vi "YKMW100 Get Error Log.vi"(0 "VISA session":refnum<visa-resource-name>="MW100", 2 "Semiphore":T1, 9 "Timeout (25000)":u32=100, 11 "error in (no error)":errorcluster, 13 "Source (\"\")":string) -> (4 "dup VISA session":refnum<visa-resource-name>, 6 "Error History":string[](array[string]), 7 "Send Message (\"\")":string, 15 "error out":errorcluster)   [LabVIEW 2009]
doc: "This VI sends the message. Then it returns the response."
panel:
  out "Read Buffer":string
  in  "Number of Read Blocks (1-50)":i32
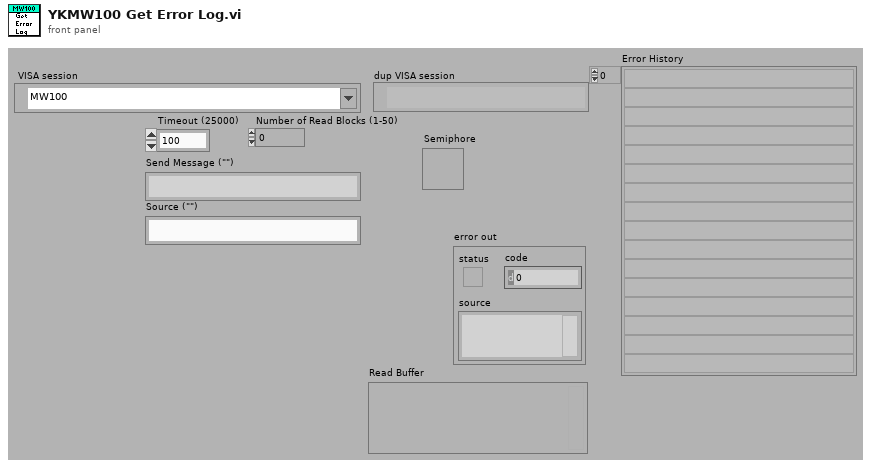
[diagram p1: front panel]
types:
  T1 = typedef "Semaphore RefNum" = refnum<k1>
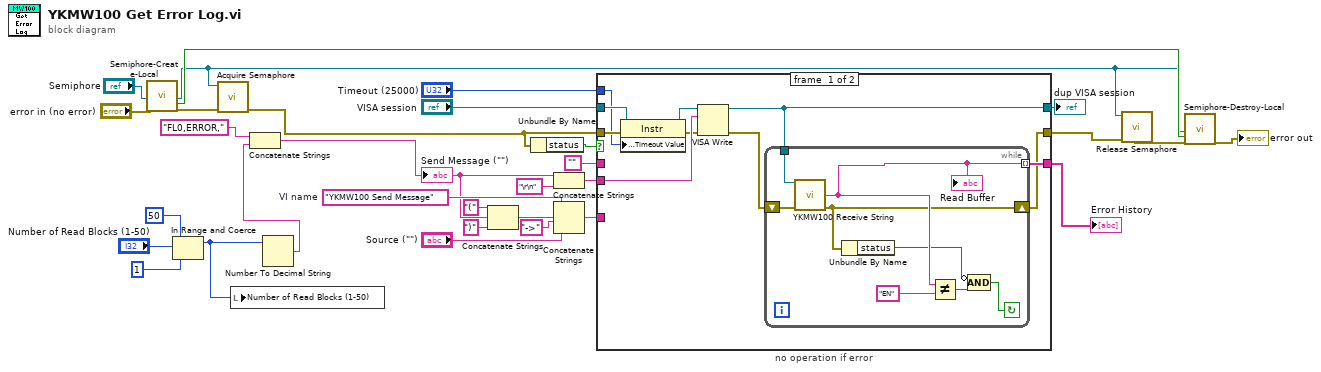
[diagram p0: block diagram]
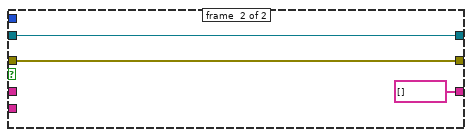
[diagram p2: hidden frame]
diagram:
  w21 = "YKMW100 Send Message"  # VI name
  n1 = call "Semiphore-Create-Local.vi"("Semiphore"="Semiphore", "error in (no error)"="error in (no error)") -> ("semaphore"=w1:T1, "Local?"=w4:bool, "error out"=w7:errorcluster)  [unwired: 15 in]
  n2 = In Range and Coerce(upper limit=50, x="Number of Read Blocks (1-50)", lower limit=1) -> (coerced(x)=w13:i32)  [unwired: 1 out]
  n3 = call <vilib>:"Acquire Semaphore.vi"("error in (no error)"=w7, "semaphore"=w1) -> ("error out"=w3:errorcluster)  [unwired: 3 in, 2 out]
  n4 = local write "Number of Read Blocks (1-50)"(w13) -> ()
  n5 = Number To Decimal String(number=w13) -> (decimal integer string=w12:string)  [unwired: 1 in]
  n6 = Concatenate Strings("FL0,ERROR,", w12) -> (w11:string)
  "Send Message (\"\")" <- w11
  n7 = Concatenate Strings("(", w11, ")") -> (w22:string)
  n8 = Unbundle By Name(w3) -> ("status"=w28:bool)
  n9 = Concatenate Strings(w11, "\r\n") -> (w31:string)
  n10 = Concatenate Strings(w21, w22, "->", "Source (\"\")") -> (w27:string)
  n11 = case "no operation if error" shown="False" w28 {
    tunnel: "VISA session" -> [w38 w52]
    tunnel: w31 -> [w41 _]
    tunnel: [w32 w52] -> w20
    tunnel: [w34 w51] -> w6
    tunnel: w3 -> [w40 w51]
    tunnel: w27 -> [_ _]
    tunnel: "Timeout (25000)" -> [w36 _]
    tunnel: [w35 string[] []] -> w10
    tunnel: "" -> [_ _]
    frame #0 {
      n12 = property class="Instr"(reference=w38, error in=w40, "General Settings:Timeout Value"=w36) -> (reference out=w37:refnum<visa-resource-name>, error out=w39:errorcluster)
      n13 = VISA Write(VISA resource name=w37, write buffer=w41, error in (no error)=w39) -> (VISA resource name out=w32:refnum<visa-resource-name>, error out=w33:errorcluster)  [unwired: 1 out]
      n14 = while {
        tunnel: w32 -> [w49]
        tunnel: [w47] -> w35 mode=indexing
        shift-right: [w43] -> w34
        shift-left: w33 -> [w48]
        stop <- w44 continue-if-true
        n15 = call "YKMW100 Receive String.vi"("VISA session"=w49, "error in (no error)"=w48) -> ("Read Buffer"=w47:string, "error out"=w43:errorcluster)  [unwired: 11 in, 1 out]
        "Read Buffer" <- w47
        n16 = Unbundle By Name(w43) -> ("status"=w45:bool)
        n17 = Not Equal?(x=w47, y="EN" ("concatenated string")) -> (x != y?=w46:bool)
        n18 = Compound Arithmetic op=AND(invert w45, w46) -> (w44:bool)
      }
    }
    frame #1 {
    }
  }
  "dup VISA session" <- w20
  "Error History" <- w10
  n19 = call <vilib>:"Release Semaphore.vi"("error in (no error)"=w6, "semaphore"=w1) -> ("error out"=w2:errorcluster)  [unwired: 4 in, 1 out]
  n20 = call "Semiphore-Destroy-Local.vi"("Semiphore"=w1, "Local?"=w4, "error in (no error)"=w2) -> ("error out"=→"error out":errorcluster)  [unwired: 16 in]
